vi "close_db.vi"(8 "error in (no error)":errorcluster, 11 "BD in":refnum<class "Base de Datos.lvclass">) -> (0 "error out":errorcluster, 3 "BD out":refnum<class "Base de Datos.lvclass">)   [LabVIEW 2019, in "Base de Datos.lvclass"]
uses:
  Base de Datos.lvclass
  Base de Datos.lvclass/Base de Datos.ctl
  SQLiteConnector/SQLiteConnection.lvclass
panel:
  # "Close DB reference"
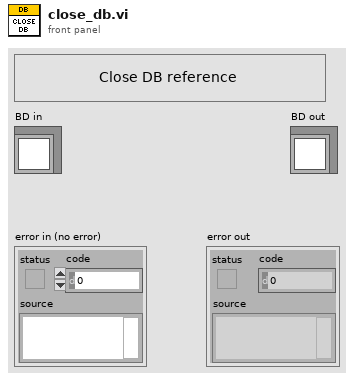
[diagram p1: front panel]
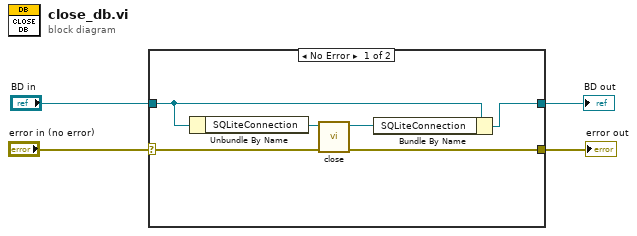
[diagram p0: block diagram]
diagram:
  n1 = case shown="No Error" "error in (no error)" {
    selector: "error in (no error)" -> [w9 w12]
    tunnel: [w10 w12] -> w4
    tunnel: "BD in" -> [w7 w11]
    tunnel: [w6 w11] -> w1
    frame No Error {
      n2 = Unbundle By Name(w7) -> ("SQLiteConnection"=w8:refnum<class "SQLiteConnection.lvclass">)
      n3 = call-dynamic "close.vi"("error in (no error)"=w9, "object in"=w8) -> ("error out"=w10:errorcluster, "object out"=w5:refnum<class "SQLiteConnection.lvclass">)  [unwired: 8 in]
      n4 = Bundle By Name(cluster=w7, "SQLiteConnection"=w5) -> (w6:refnum<class "Base de Datos.lvclass">)
    }
    frame Error {
    }
  }
  "error out" <- w4
  "BD out" <- w1
